vi "Error Handler and Log.vi"(8 "error in (no error)":errorcluster, 10 "Current Bus Number":i32, 11 "Queue in":refnum<queue>) -> (0 "error out":errorcluster, 1 "error out (maintain error)":errorcluster, 2 "Current Status":string, 3 "Queue out":refnum<queue>, 5 "Next State":T1)   [LabVIEW 2014, in "SPI Engine Scripting.lvlib"]
doc: "Handles errors and creates the Current Status entry for the Scripting Log. Errors will be printed to the log if they occur and will cause the scripting sequence to go to the End state."
uses:
  SPI Engine Scripting.lvlib
  Scripting States.ctl
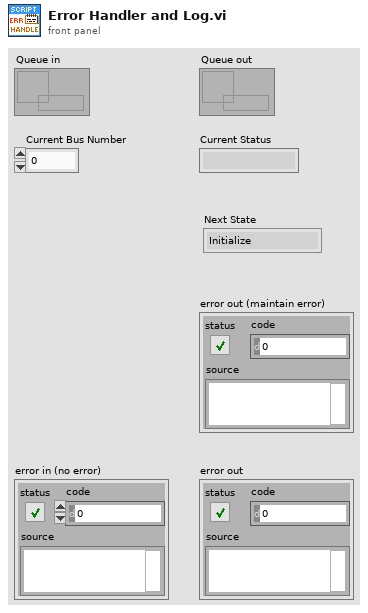
[diagram p1: front panel]
types:
  T1 = typedef "Scripting States.ctl" = enum16{"Initialize", "Copy Template Bus Directory", "Modify Dequeue Commands", "Modify Enqueue Data", "Create FPGA VI", "Create Project FIFOs", "Create FPGA Data Nodes", "Place FPGA Data Nodes", "Update Node Count in Engine", "Expand FIFO Type Def", "Populate FIFO Names in Engine", "Modify I/O Pin Names", "Modify I/O Pin Enable", "Replace DLU", "Add Engine to Project", "Place SPI Engine", "Scripting Complete Check", "End"}
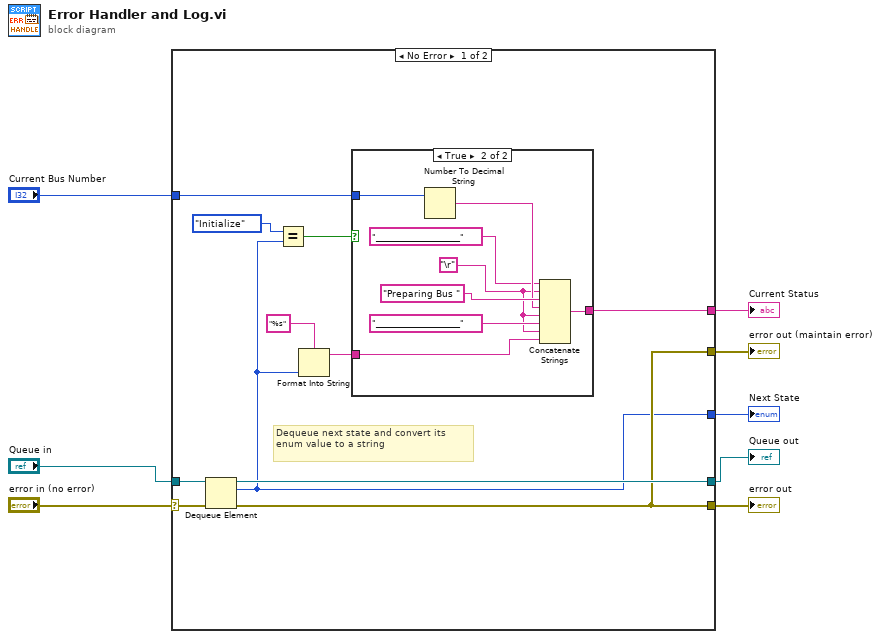
[diagram p0: block diagram]
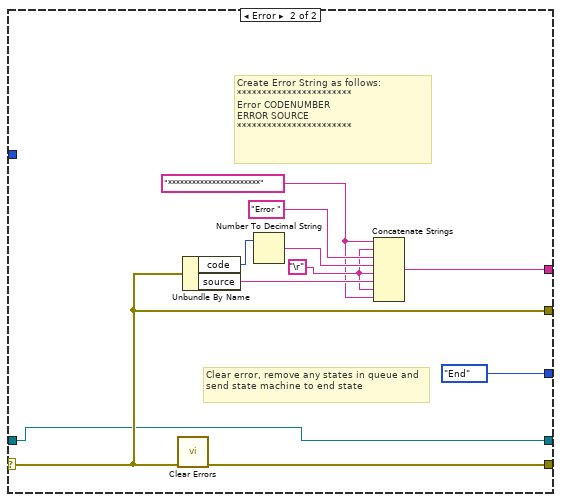
[diagram p3: hidden frame]
diagram:
  n1 = case shown="No Error" "error in (no error)" {
    selector: "error in (no error)" -> [w19 w32]
    tunnel: [w12 w36] -> w2
    tunnel: "Queue in" -> [w18 w31]
    tunnel: [w10 w30] -> w7
    tunnel: [w17 w31] -> w8
    tunnel: "Current Bus Number" -> [w14 _]
    tunnel: [w10 w32] -> w6
    tunnel: [w9 Scripting_States."End"] -> w1
    frame No Error {
      # "Dequeue next state and convert its enum value to a string"
      n2 = Dequeue Element(queue=w18, error in (no error)=w19) -> (queue out=w17:refnum<queue>, element=w9:T1, error out=w10:errorcluster)  [unwired: 1 in, 1 out]
      n3 = Equal?(x=Scripting_States."Initialize" ("element"), y=w9) -> (x = y?=w13:bool)
      n4 = Format Into String "Format Into String"(format string="%s", w9) -> (resulting string=w11:string)  [unwired: 2 in, 1 out]
      n5 = case shown="True" w13 {
        tunnel: w14 -> [_ w28]
        tunnel: [w20 w27] -> w12
        tunnel: w11 -> [w20 w22]
        frame False {
        }
        frame True {
          w21 = "\r"
          n6 = Number To Decimal String(number=w28) -> (decimal integer string=w25:string)  [unwired: 1 in]
          n7 = Concatenate Strings("_____________________" ("string"), w21, "Preparing Bus " ("string"), w25, w21, "_____________________" ("string"), w21, w22) -> (w27:string)
        }
      }
    }
    frame Error {
      w33 = "***********************" ("string")
      w34 = "\r"
      # "Create Error String as follows:\n***********************\nError CODENUMBER\nERROR SOURCE\n***********************"
      # "Clear error, remove any states in queue and send state machine to end state"
      n8 = call <vilib>:"Clear Errors.vi"("error in (no error)"=w32) -> ("error out"=w30:errorcluster)  [unwired: 5 in, 1 out]
      n9 = Unbundle By Name(w32) -> ("code"=w37:i32, "source"=w39:string)
      n10 = Number To Decimal String(number=w37) -> (decimal integer string=w38:string)  [unwired: 1 in]
      n11 = Concatenate Strings(w33, w34, "Error " ("string"), w38, w34, w39, w34, w33) -> (w36:string)
    }
  }
  "Queue out" <- w8
  "error out" <- w7
  "Current Status" <- w2
  "error out (maintain error)" <- w6
  "Next State" <- w1
